vi "14_StartStop_UI.vi"(8 "error in (no error)":errorcluster) -> (0 "error out":errorcluster)   [LabVIEW 2014]
uses:
  SwabianInstruments.TimeTagger
panel:
  in  "clear":bool
  in  "binwidth":i64=1
  in  "Test signal":bool
  in  "Start channel":i32=2
  in  "Stop channel":i32=1
  in  "stop":bool
  out "StartStop Histogram":cluster{i64[], i64[]}(graph)
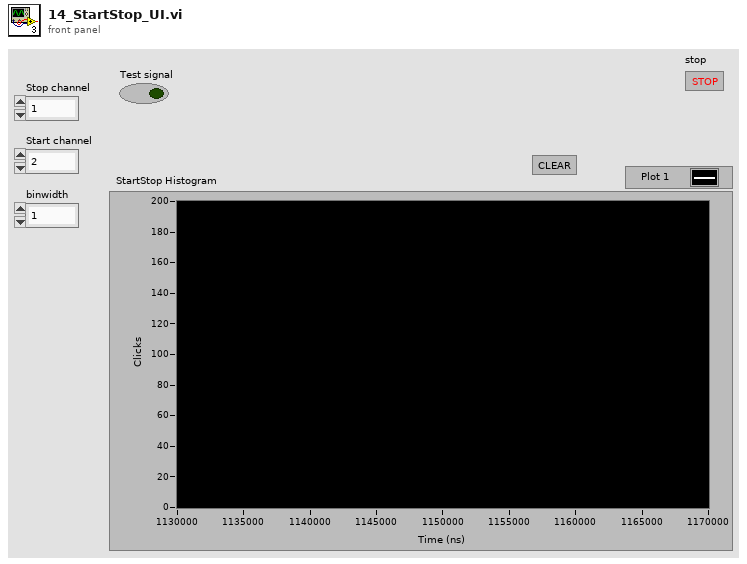
[diagram p1: front panel]
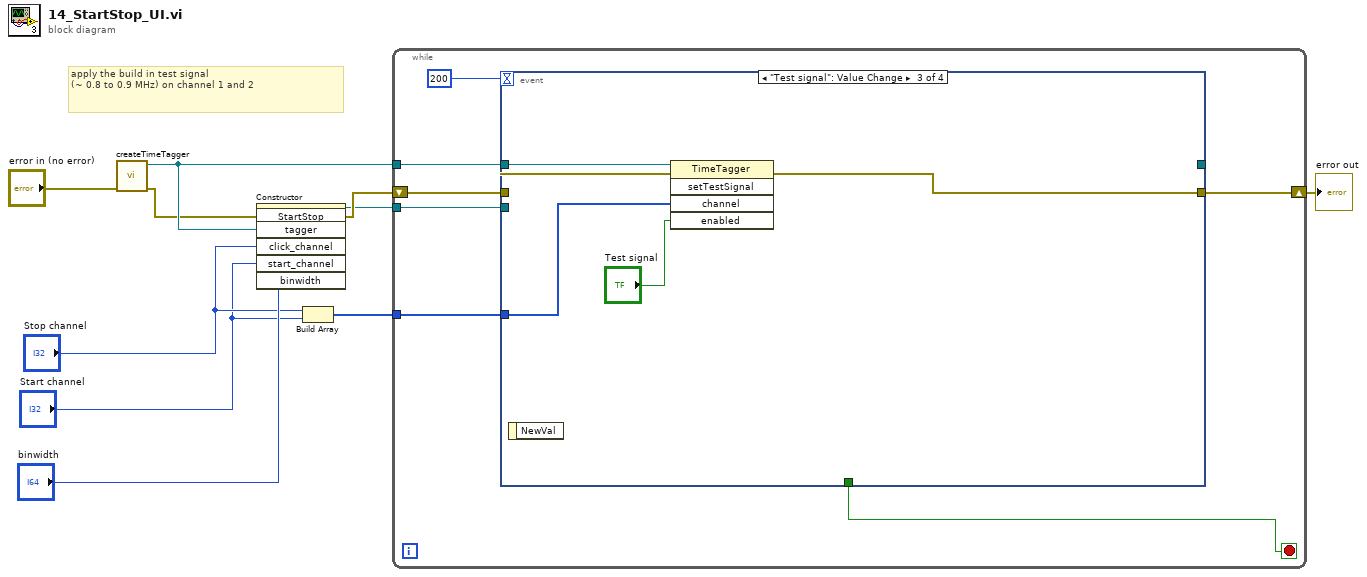
[diagram p0: block diagram]
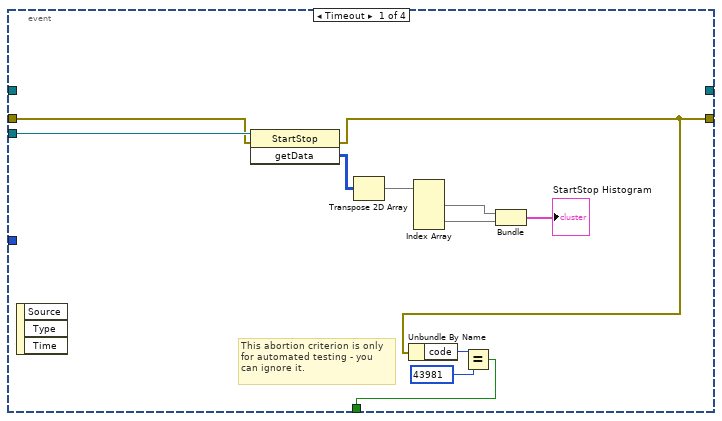
[diagram p2: hidden frame]
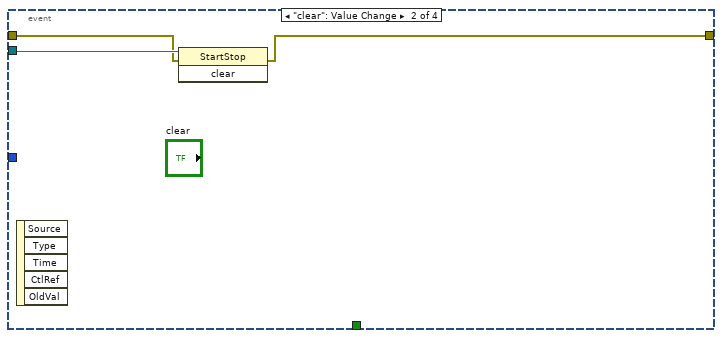
[diagram p3: hidden frame]
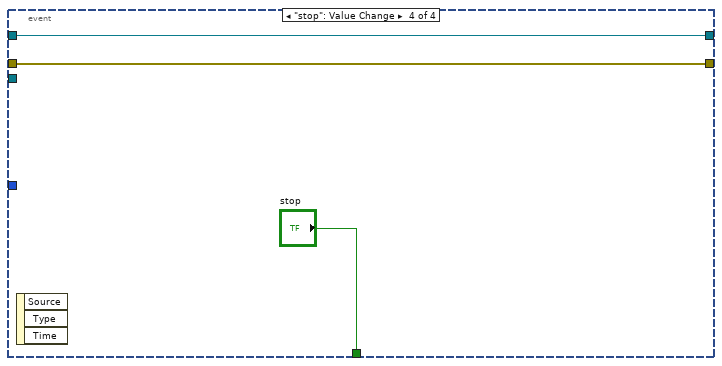
[diagram p4: hidden frame]
diagram:
  # "apply the build in test signal\n(~ 0.8 to 0.9 MHz) on channel 1 and 2"
  n1 = call "createTimeTagger.vi"("error in (no error)"="error in (no error)") -> ("error out"=w1:errorcluster, "TimeTagger ref out"=w2:refnum<k24>)  [unwired: 9 in]
  n2 = constructor class="StartStop"(error in=w1, "tagger"=w2, "click_channel"="Stop channel", "start_channel"="Start channel", "binwidth"="binwidth") -> (reference out=w9:refnum<k24>, error out=w10:errorcluster)  [unwired: 2 in, 5 out]
  n3 = Build Array("Stop channel", "Start channel") -> (w5:i32[])
  n4 = while {
    tunnel: w2 -> [w16]
    shift-right: [w15] -> w3
    shift-left: w10 -> [w17]
    tunnel: w9 -> [w14]
    tunnel: w5 -> [w12]
    stop <- w11 stop-if-true
    n5 = event shown="[2] \"Test signal\": Value Change" {
      selector: _ -> [_ _ _ _]
      dyn-events: _ -> [_ _ _ _]
      timeout: 200 -> [_ _ _ _]
      tunnel: w17 -> [w26 w30 w35 w38]
      tunnel: w16 -> [_ _ w36 w37]
      tunnel: [w19 w29 w32 w38] -> w15
      tunnel: [_ _ _ w37] -> _
      tunnel: w14 -> [w27 w31 _ _]
      tunnel: w12 -> [_ _ w33 _]
      tunnel: [w18 _ _ "stop"] -> w11
      event Timeout {
        # "This abortion criterion is only\nfor automated testing - you\ncan ignore it."
        n6 = event-data() -> ()  [unwired: 1 in, 3 out]
        n7 = invoke class="StartStop" method="getData"(reference=w27, error in=w26) -> (error out=w19:errorcluster, "getData"=w23:i64[][])  [unwired: 1 in, 1 out]
        n8 = Transpose 2D Array(2D array=w23) -> (transposed array=w22:i64[][])
        n9 = Unbundle By Name(w19) -> ("code"=w21:i32)
        n10 = Index Array(array=w22) -> (element #1=w25:i64[], element #2=w24:i64[])  [unwired: 4 in]
        n11 = Equal?(x=w21, y=43981) -> (x = y?=w18:bool)
        n12 = Bundle(w25, w24) -> (→"StartStop Histogram":cluster{i64[], i64[]})  [unwired: 1 in]
      }
      event "clear": Value Change {
        n13 = event-data() -> ()  [unwired: 1 in, 5 out]
        n14 = invoke class="StartStop" method="clear"(reference=w31, error in=w30) -> (error out=w29:errorcluster)  [unwired: 1 in, 2 out]
      }
      event "Test signal": Value Change {
        n15 = event-data() -> ()  [unwired: 1 in, 1 out]
        n16 = invoke class="TimeTagger" method="setTestSignal"(reference=w36, error in=w35, "channel"=w33, "enabled"="Test signal") -> (error out=w32:errorcluster)  [unwired: 1 in, 4 out]
      }
      event "stop": Value Change {
        n17 = event-data() -> ()  [unwired: 1 in, 3 out]
      }
    }
  }
  "error out" <- w3
